vi "projet_labview_exo1v3.vi"() -> ()   [LabVIEW 2023]
panel:
  out "blue output test":string
  out "green output test":string
  out "red output test":string
  in  "markershape":string
  in  "markersize":string
  out "Colours":u32[](array[colorbox])
  out "b 3":u8[](array[numeric])
  out "g 2":u8[](array[numeric])
  out "r":u8[](array[numeric])
  out "clut":u32[](array[numeric])
  out "matlabium filename test":string
  out "filename":string
  out "output matlab":string
  out "MATLABIUM":string
  out "error out 2":errorcluster
  out "Tracestxt":string
  out "standard error":string
  out "standard output":string
  out "Scanned Image":picture
  in  "Path":path
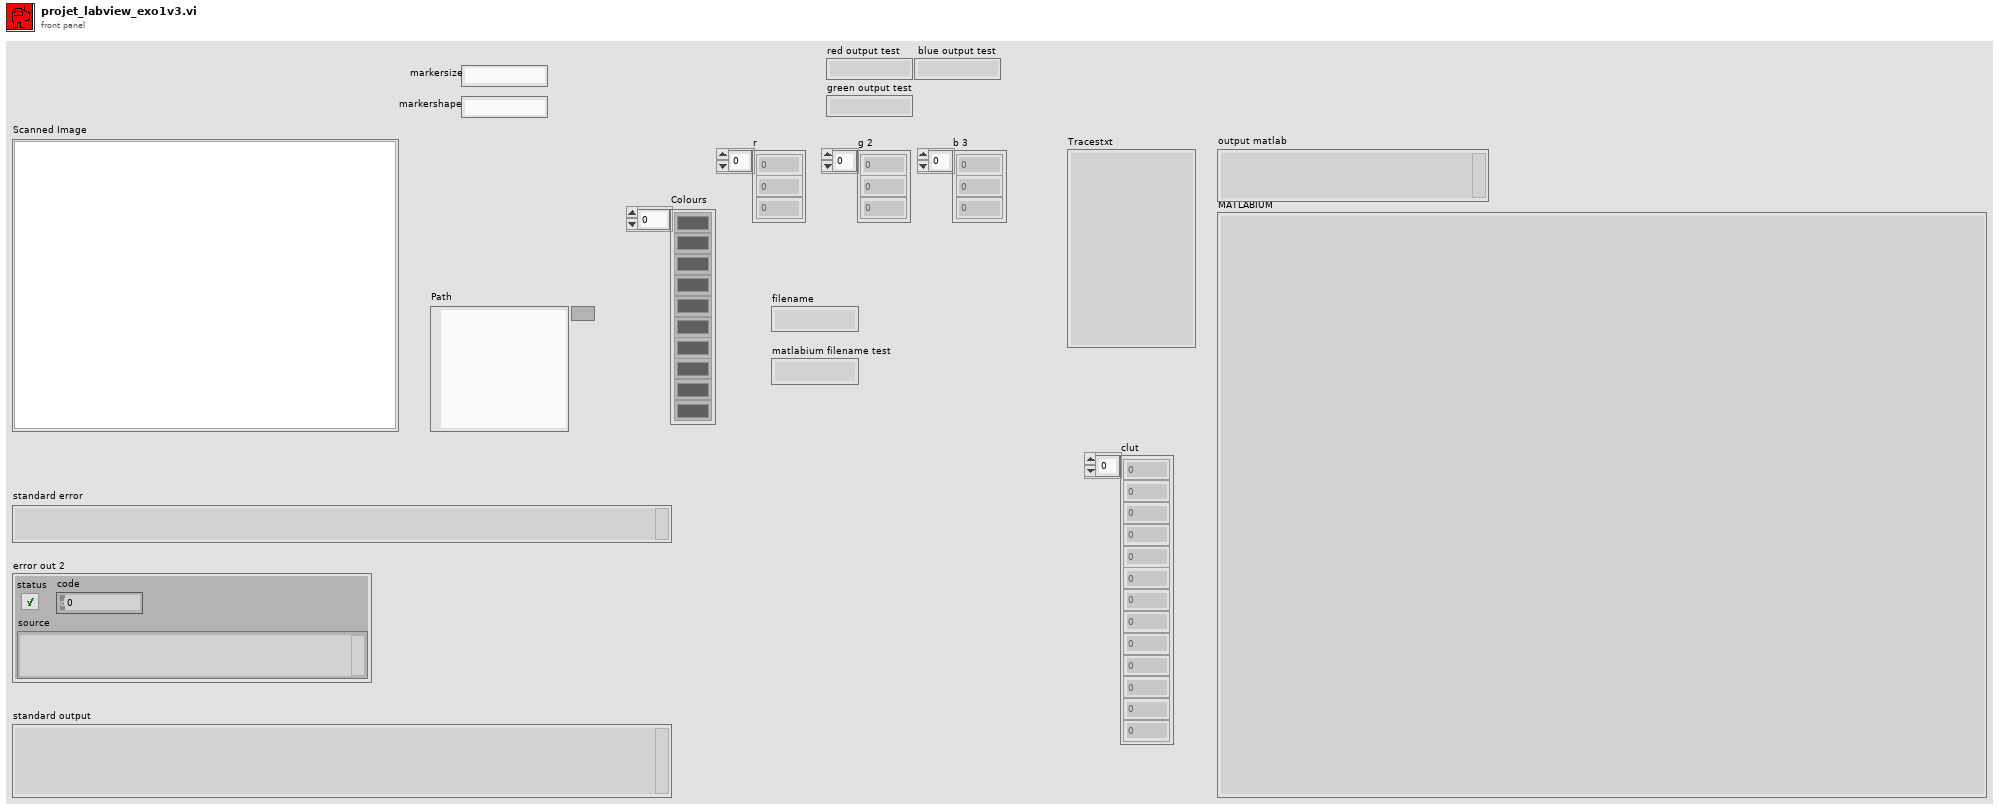
[diagram p1: front panel]
types:
  T1 = enum16{"big-endian, network order", "native, host order", "little-endian"}
  T2 = typedef "imagedata.ctl" = cluster{"image type":i32, "image depth":i32, "image":u8[], "mask":u8[], "colors":u32[], "Rectangle":cluster{"left":i16, "top":i16, "right":i16, "bottom":i16}}
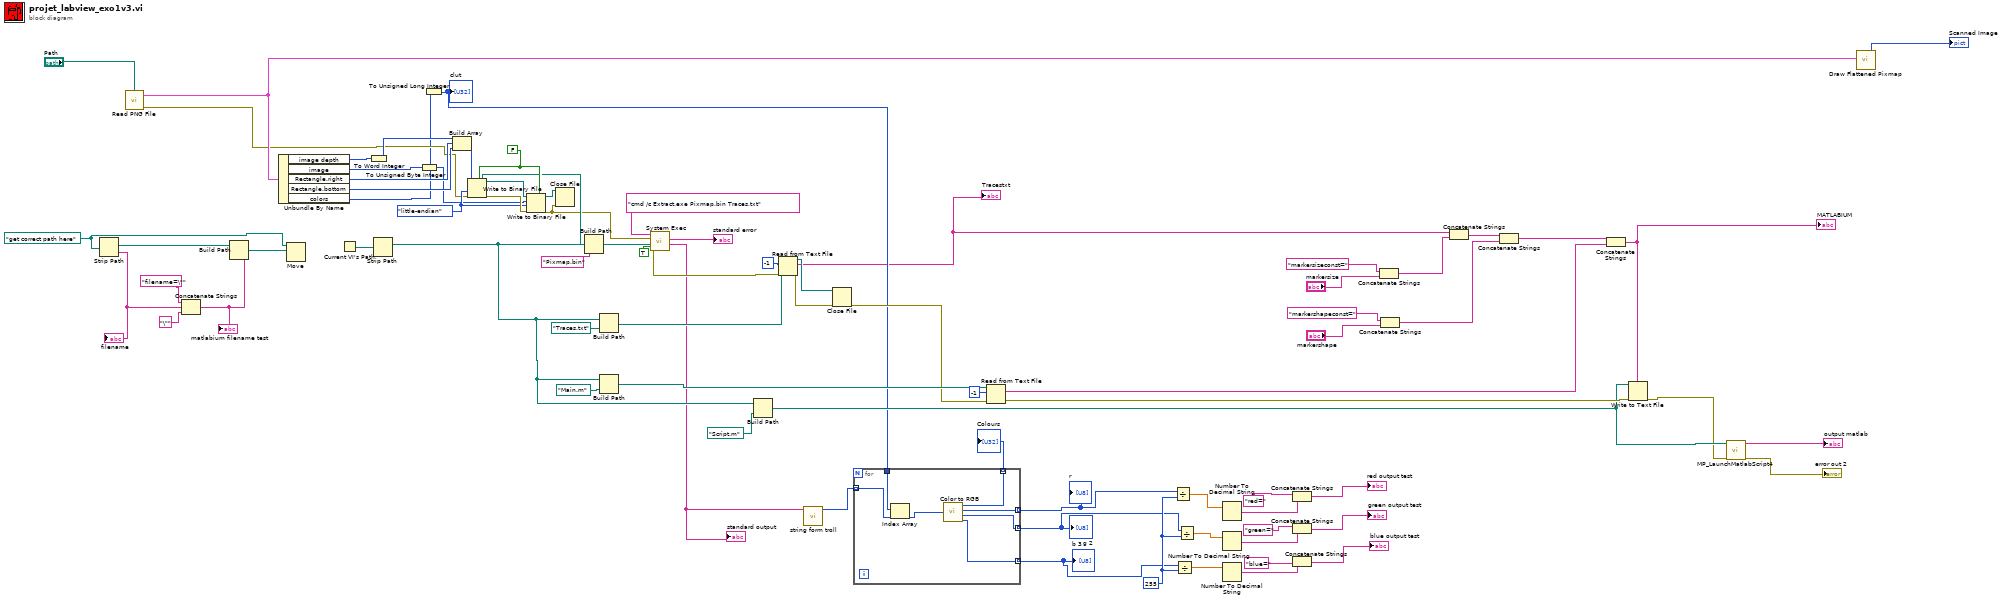
[diagram p0: block diagram]
diagram:
  w1 = path "get correct path here"
  w23 = 255
  w68 = T1."little-endian" ("byte order (0:big-endian, network order)")
  w74 = FALSE
  n1 = Strip Path(path=w1) -> (stripped path=w4:path, name=w39:string)
  "filename" <- w39
  n2 = call <vilib>:"Read PNG File.vi"("path to PNG file"="Path") -> ("error out"=w53:errorcluster, "image data"=w72:T2)  [unwired: 8 in, 1 out]
  n3 = Concatenate Strings("filename=\"" ("string"), w39, "\"" ("string")) -> (w8:string)
  "matlabium filename test" <- w8
  n4 = Build Path(base path=w4, name or relative path=w8) -> (appended path=w2:path)
  n5 = Unbundle By Name(w72) -> ("image depth"=w77:i32, "image"=w36:u8[], "Rectangle.right"=w76:i16, "Rectangle.bottom"=w75:i16, "colors"=w35:u32[])
  n6 = Move(source path=w1, 10:w2) -> ()  [unwired: 3 in, 3 out]
  n7 = Current VI's Path() -> (path=w66:path)
  n8 = To Word Integer(number=w77) -> (16bit integer=w78:i16)
  n9 = Strip Path(path=w66) -> (stripped path=w46:path)  [unwired: 1 out]
  n10 = To Unsigned Byte Integer(number=w36) -> (unsigned 8bit integer=w61:u8[])
  n11 = To Unsigned Long Integer(number=w35) -> (unsigned 32bit integer=w34:u32[])
  "clut" <- w34
  n12 = Build Array(w78, w76, w75) -> (w62:i16[])
  n13 = Build Path(base path=w46, name or relative path="Pixmap.bin" ("String")) -> (appended path=w67:path)
  n14 = Write to Binary File(file (use dialog)=w67, data=w62, error in=w53, 5:w74, 9:w68) -> (refnum out=w60:refnum<file>, error out=w73:errorcluster)  [unwired: 1 in, 1 out]
  n15 = Write to Binary File(file (use dialog)=w60, data=w61, error in=w73, 5:w74, 9:w68) -> (refnum out=w63:refnum<file>, error out=w64:errorcluster)  [unwired: 1 in, 1 out]
  n16 = Close File(refnum=w63, error in=w64) -> ()  [unwired: 2 out]
  n17 = Build Path(base path=w46, name or relative path=path "Traces.txt") -> (appended path=w58:path)
  n18 = Build Path(base path=w46, name or relative path=path "Main.m") -> (appended path=w51:path)
  n19 = call <vilib>:"System Exec.vi"("run minimized? (F)"=TRUE, "error in (no error)"=w64, "working directory"=w46, "command line"="cmd /c Extract.exe Pixmap.bin Traces.txt") -> ("error out"=w57:errorcluster, "standard error"=→"standard error":string, "standard output"=w33:string)  [unwired: 4 in, 1 out]
  "standard output" <- w33
  n20 = Build Path(base path=w46, name or relative path=path "Script.m") -> (appended path=w44:path)
  n21 = Read from Text File(file (use dialog)=w58, count=-1, error in=w57) -> (refnum out=w55:refnum<file>, text=w30:string, error out=w54:errorcluster)  [unwired: 1 in, 1 out]
  "Tracestxt" <- w30
  n22 = call "string form troll.vi"("String"=w33) -> ("Array"=w32:u32[])  [unwired: 10 in]
  n23 = Close File(refnum=w55, error in=w54) -> (error out=w50:errorcluster)  [unwired: 1 out]
  n24 = for {
    tunnel: w32 -> [w86] mode=indexing
    tunnel: w34 -> [w85]
    tunnel: [w84] -> w24 mode=indexing
    tunnel: [w83] -> w21 mode=indexing
    tunnel: [w82] -> w22 mode=indexing
    tunnel: [w80] -> w31 mode=indexing
    n25 = Index Array(array=w85, index=w86) -> (element=w81:u32)
    n26 = call <vilib>:"Color to RGB.vi"("Color"=w81) -> ("Resolved Color"=w80:u32, "R"=w84:u8, "G"=w83:u8, "B"=w82:u8)
  }
  "r" <- w24
  "g 2" <- w21
  "b 3" <- w22
  "Colours" <- w31
  n27 = Read from Text File(file (use dialog)=w51, count=-1, error in=w50) -> (text=w40:string, error out=w47:errorcluster)  [unwired: 1 in, 2 out]
  n28 = Divide(x=w24, y=w23) -> (x/y=w20:dbl[])
  n29 = Divide(x=w22, y=w23) -> (x/y=w18:dbl[])
  n30 = Divide(x=w21, y=w23) -> (x/y=w19:dbl[])
  n31 = Number To Decimal String(number=w20) -> (decimal integer string=w11:string[])  [unwired: 1 in]
  n32 = Number To Decimal String(number=w19) -> (decimal integer string=w10:string[])  [unwired: 1 in]
  n33 = Number To Decimal String(number=w18) -> (decimal integer string=w9:string[])  [unwired: 1 in]
  n34 = Concatenate Strings("red=", w11) -> (→"red output test":string)
  n35 = Concatenate Strings("green=", w10) -> (→"green output test":string)
  n36 = Concatenate Strings("blue=", w9) -> (→"blue output test":string)
  n37 = Concatenate Strings("markersizeconst=", "markersize") -> (w25:string)
  n38 = Concatenate Strings("markershapeconst=", "markershape") -> (w15:string)
  n39 = Concatenate Strings(w30, w25) -> (w16:string)
  n40 = Concatenate Strings(w16, w15) -> (w17:string)
  n41 = Concatenate Strings(w17, w40) -> (w48:string)
  "MATLABIUM" <- w48
  n42 = Write to Text File(file (use dialog)=w44, text=w48, error in=w47) -> (error out=w42:errorcluster)  [unwired: 1 in, 2 out]
  n43 = call "MP_LaunchMatlabScript4.vi"("error in (no error)"=w42, "matlab script path"=w44) -> ("error out"=→"error out 2":errorcluster, "standard output"=→"output matlab":string)  [unwired: 4 in, 4 out]
  n44 = call <vilib>:"Draw Flattened Pixmap.vi"("image data"=w72) -> ("new picture"=→"Scanned Image":picture)  [unwired: 8 in]
